vi "Run.vi"(8 "error in (no error)":errorcluster, 9 "Time Ratio used":dbl, 10 "Maze (0: Empty, -1: Enemy. >0: Teammate":i32[][](array[numeric]), 11 "Line Dancer in":refnum<class "Bricks.lvclass">) -> (0 "error out":errorcluster, 1 "Direction":T1, 2 "Action":T2, 3 "Line Dancer out":refnum<class "Bricks.lvclass">, 4 "Replicated":refnum<class "Square.lvclass">)   [LabVIEW 2015, in "Bricks.lvclass"]
uses:
  Bricks.lvclass
  Type Defs/Action Enum.ctl
  Type Defs/Direction Enum.ctl
  Square/Square.lvclass
  Common/Position.ctl
  Bricks.lvclass/Bricks.ctl
  Brick Wall Type.ctl
  SubVIs/Read-Only Globals.vi
  Common/Reverse Direction.vi
  Type Defs/SB Type Defs.lvlib
  Common/Common.lvlib
panel:
  # "NOTICE - YOU MUST NOT REMOVE THIS NOTICE. PER THE FOLLOWING LICENSE, YOU MAY REPRODUCE THIS SOFTWARE PROVIDED YOU FOLLOW THE TERMS\nOF THE LICENSE.\n\n---BEGIN BSD LICENSE (http://opensource.org/licenses/BSD-2-Clause)---\nCopyright (c) 2015, Endigit, Inc. <robert@endigit.com>\nAll rights reserved.\n\nRedistribution and use in source and binary forms, with or without modification, are permitted provided that the following conditions are met:\n\n1. Redistributions of source code must retain the above copyright notice, this list of conditions and the following disclaimer.\n\n2. Redistributions in binary form must reproduce the above copyright notice, this list of conditions and the following disclaimer in the documentation and/or other \nmaterials provided with the distribution.\n\nTHIS SOFTWARE IS PROVIDED BY THE COPYRIGHT HOLDERS AND CONTRIBUTORS \"AS IS\" AND ANY EXPRESS OR IMPLIED WARRANTIES, INCLUDING, BUT NOT \nLIMITED TO, THE IMPLIED WARRANTIES OF MERCHANTABILITY AND FITNESS FOR A PARTICULAR PURPOSE ARE DISCLAIMED. IN NO EVENT SHALL THE COPYRIGHT \nHOLDER OR CONTRIBUTORS BE LIABLE FOR ANY DIRECT, INDIRECT, INCIDENTAL, SPECIAL, EXEMPLARY, OR CONSEQUENTIAL DAMAGES (INCLUDING, BUT NOT \nLIMITED TO, PROCUREMENT OF SUBSTITUTE GOODS OR SERVICES; LOSS OF USE, DATA, OR PROFITS; OR BUSINESS INTERRUPTION) HOWEVER CAUSED AND ON \nANY THEORY OF LIABILITY, WHETHER IN CONTRACT, STRICT LIABILITY, OR TORT (INCLUDING NEGLIGENCE OR OTHERWISE) ARISING IN ANY WAY OUT OF THE USE \nOF THIS SOFTWARE, EVEN IF ADVISED OF THE POSSIBILITY OF SUCH DAMAGE.\n---END BSD LICENSE---"
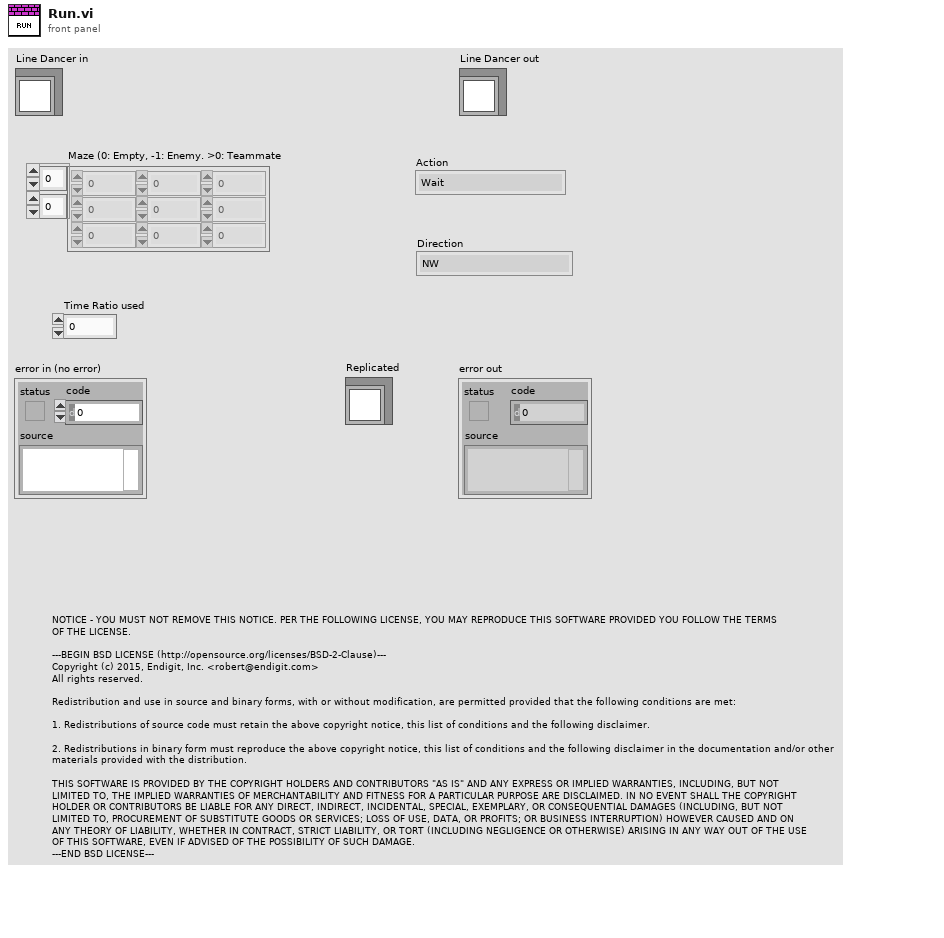
[diagram p1: front panel]
types:
  T1 = typedef "SB Type Defs.lvlib/Direction Enum.ctl" = enum16{"NW", "N", "NE", "E", "SE", "S", "SW", "W"}
  T2 = typedef "SB Type Defs.lvlib/Action Enum.ctl" = enum16{"Wait", "Move", "Attack", "Replicate"}
  T3 = typedef "Common.lvlib/Position.ctl" = cluster{"Column":i32, "Row":i32}
  T4 = typedef "Bricks.lvclass/Brick Wall Type.ctl" = enum16{"Starter", "Spawner", "Mason", "Wall", "Hottie"}
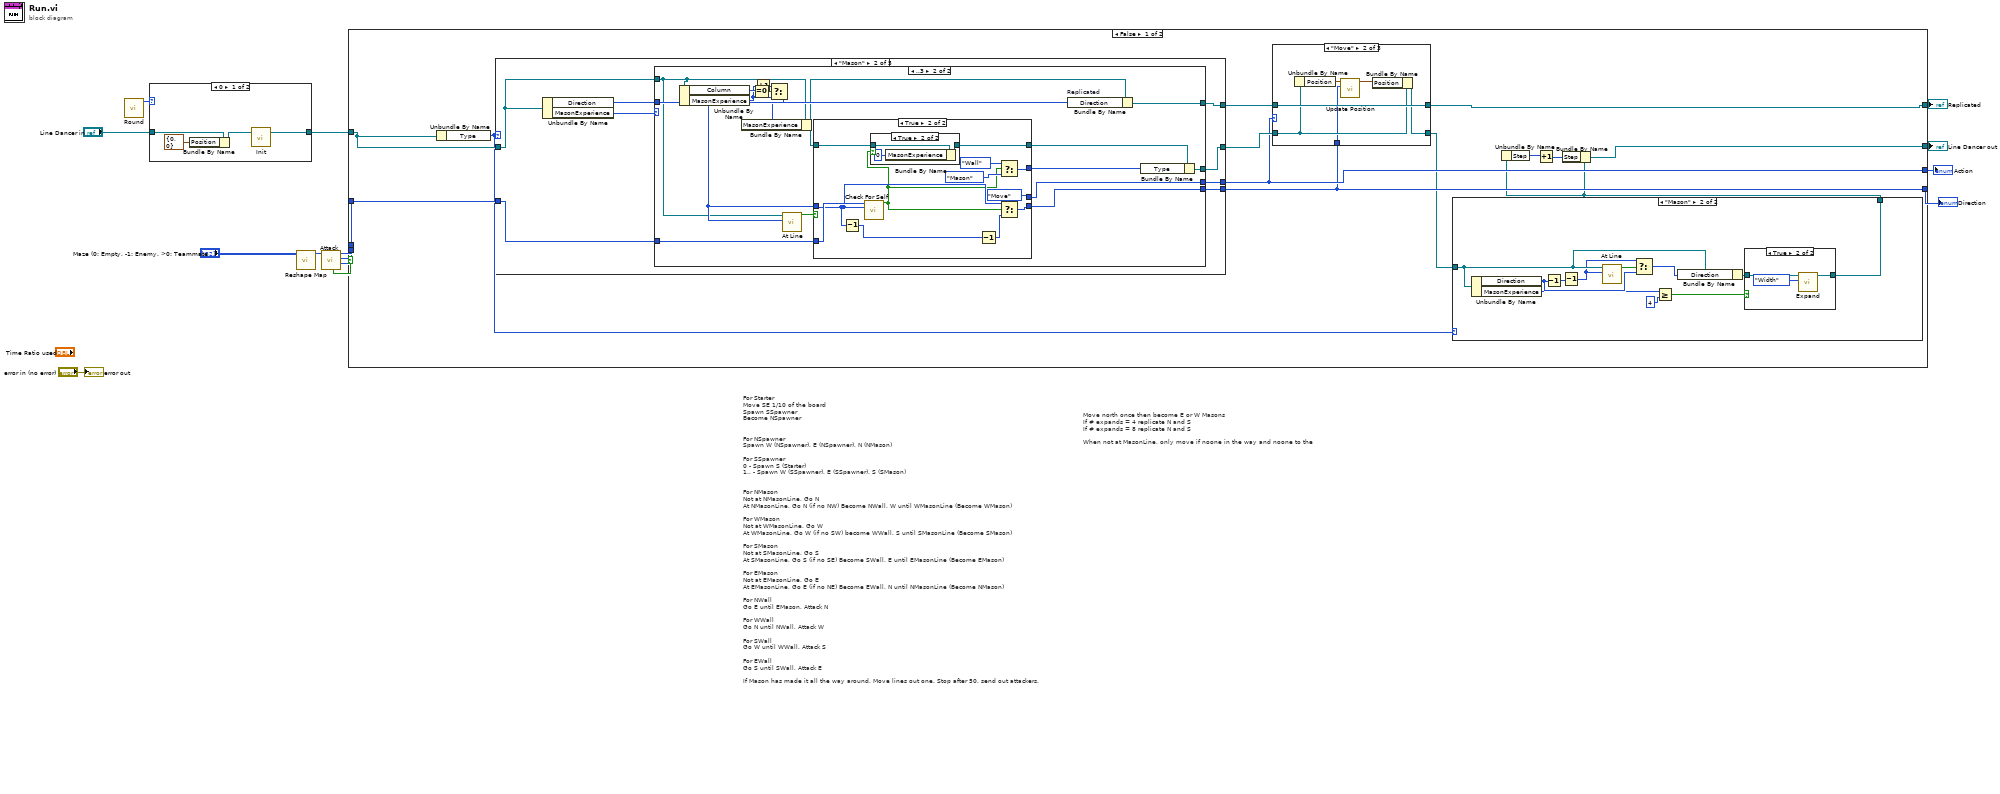
[diagram p0: block diagram]
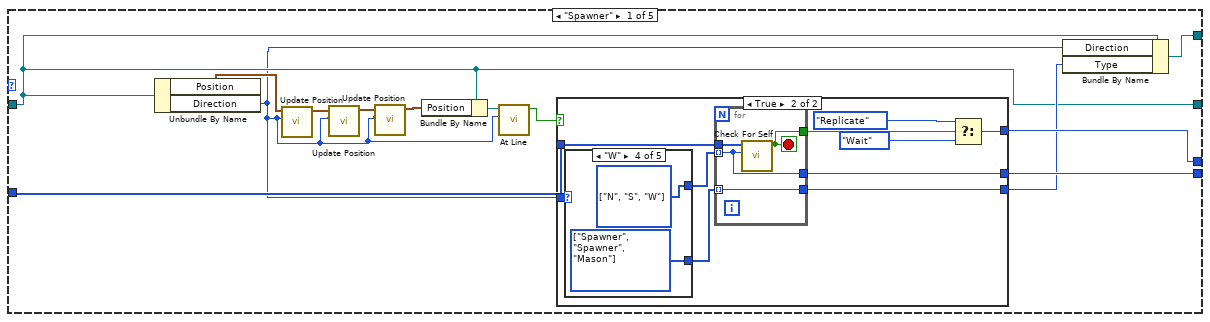
[diagram p5: hidden frame]
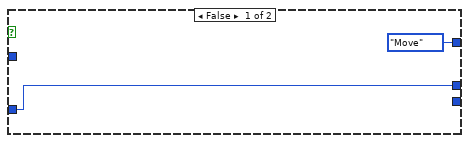
[diagram p6: hidden frame]
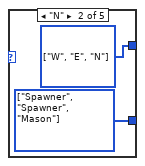
[diagram p8: hidden frame]
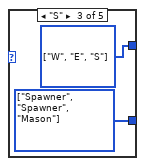
[diagram p9: hidden frame]
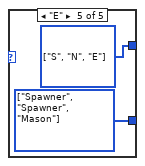
[diagram p10: hidden frame]
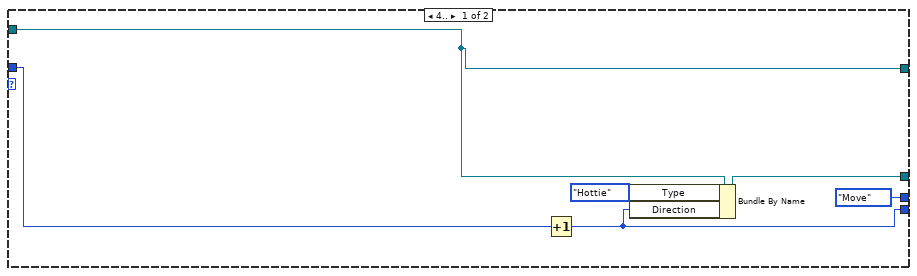
[diagram p11: hidden frame]
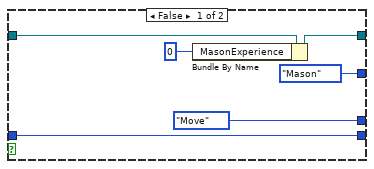
[diagram p12: hidden frame]
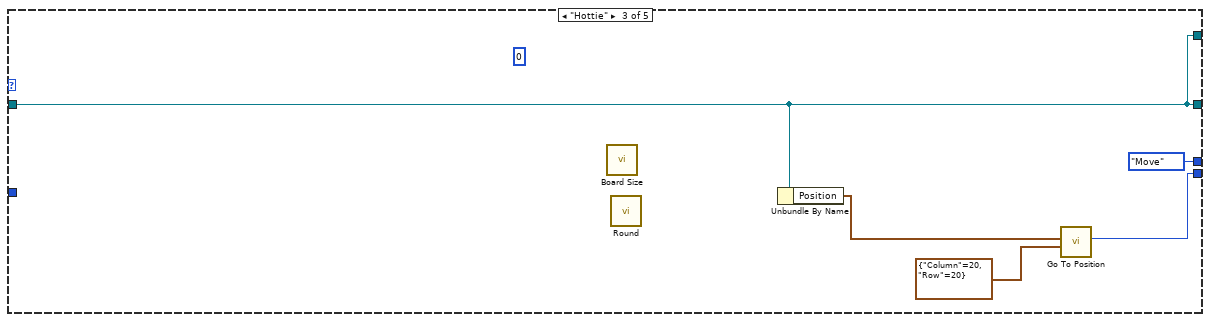
[diagram p14: hidden frame]
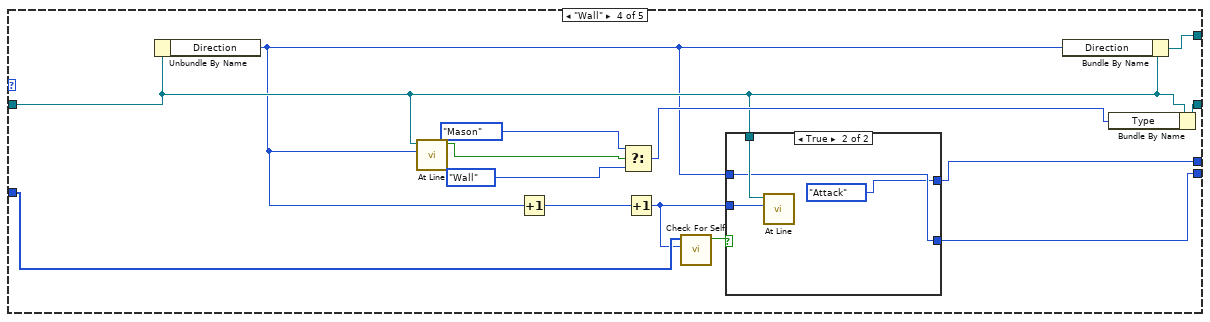
[diagram p15: hidden frame]
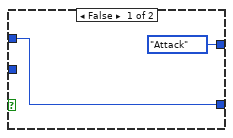
[diagram p16: hidden frame]
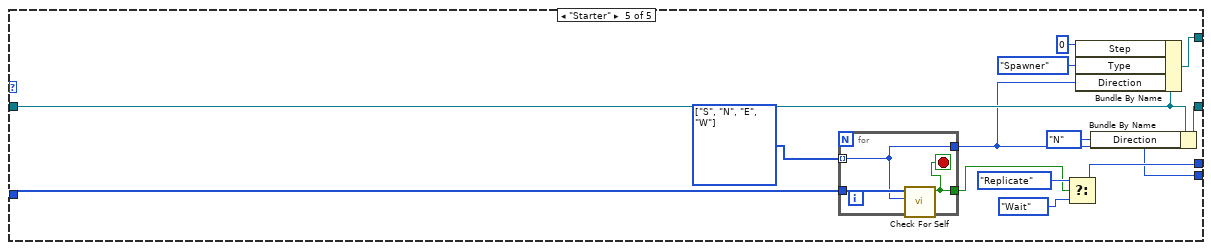
[diagram p17: hidden frame]
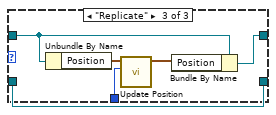
[diagram p19: hidden frame]
diagram:
  # "Move north once then become E or W Masons\nIf # expands = 4 replicate N and S\nIf # expands = 8 replicate N and S\n\nWhen not at MasonLine, only move if noone in the way and noone to the"
  # "For Starter \nMove SE 1/10 of the board\nSpawn SSpawner\nBecome NSpawner\n\n\nFor NSpawner\nSpawn W (NSpawner), E (NSpawner), N (NMason)\n\nFor SSpawner\n0 - Spawn S (Starter)\n1.. - Spawn W (SSpawner), E (SSpawner), S (SMason)\n\n\nFor NMason\nNot at NMasonLine, Go N\nAt NMasonLine, Go N (if no NW) Become NWall, W until WMasonLine (Become WMason)\n\nFor WMason\nNot at WMasonLine, Go W\nAt WMasonLine, Go W (if no SW) become WWall, S until SMasonLine (Become SMason)\n\nFor SMason\nNot at SMasonLine, Go S\nAt SMasonLine, Go S (if no SE) Become SWall, E until EMasonLine (Become EMason)\n\nFor EMason\nNot at EMasonLine, Go E\nAt EMasonLine, Go E (if no NE) Become EWall, N until NMasonLine (Become NMason)\n\nFor NWall\nGo E until EMason, Attack N\n\nFor WWall\nGo N until NWall, Attack W\n\nFor SWall\nGo W until WWall, Attack S\n\nFor EWall\nGo S until SWall, Attack E\n\nIf Mason has made it all the way around, Move lines out one. Stop after 50, send out attackers."
  n1 = call "Round.vi"() -> ("Round"=w1:i32)  [unwired: 11 in]
  n2 = case shown="0" w1 {
    tunnel: "Line Dancer in" -> [w18 w19]
    tunnel: [w17 w19] -> w2
    frame 0 {
      n3 = Bundle By Name(cluster=w18, "Position"=T3 {"Column"=0, "Row"=0}) -> (w16:refnum<class "Bricks.lvclass">)
      n4 = call "Init.vi"("Bricks in"=w16) -> ("Bricks out"=w17:refnum<class "Bricks.lvclass">)  [unwired: 10 in]
    }
    frame Default {
    }
  }
  n5 = call "Reshape Map.vi"("Maze (0: Empty, -1: Enemy. >0: Teammate"="Maze (0: Empty, -1: Enemy. >0: Teammate") -> ("Map"=w9:i32[])  [unwired: 9 in, 1 out]
  n6 = call "Attack.vi"("Maze (0: Empty, -1: Enemy. >0: Teammate"=w9) -> ("Direction"=w4:i32, "Action"=w5:T2, "Maze (0: Empty, -1: Enemy. >0: Teammate 2"=w7:i32[], "Enemy Found?"=w6:bool)  [unwired: 5 in, 2 out]
  n7 = case shown="False" w6 {
    tunnel: [w26 w194] -> w13
    tunnel: [w25 w193] -> w12
    tunnel: w2 -> [w32 w195]
    tunnel: [w29 w195] -> w11
    tunnel: [w20 w195] -> w10
    tunnel: w7 -> [w24 _]
    tunnel: w5 -> [_ w194]
    tunnel: w4 -> [_ w193]
    frame False {
      n8 = Unbundle By Name(w32) -> ("Type"=w23:T4)
      n9 = case shown="\"Mason\"" w23 {
        tunnel: [w59 w92 Action_Enum."Move" ("f") w148 w171] -> w26
        tunnel: [w60 w91 w138 w144 w167] -> w25
        tunnel: w24 -> [w61 w90 _ w147 w172]
        tunnel: [w58 w93 w141 w156 w174] -> w28
        tunnel: [w53 w89 w141 w154 w164] -> w27
        tunnel: w32 -> [w53 w87 w141 w150 w170]
        frame "Spawner" {
          n10 = Unbundle By Name(w53) -> ("Position"=w56:T3, "Direction"=w50:T1)
          n11 = call "Update Position.vi"("Direction"=w50, "Position in"=w56) -> ("Position out"=w55:T3)  [unwired: 9 in]
          n12 = call "Update Position.vi"("Direction"=w50, "Position in"=w55) -> ("Position out"=w54:T3)  [unwired: 9 in]
          n13 = call "Update Position.vi"("Direction"=w50, "Position in"=w54) -> ("Position out"=w51:T3)  [unwired: 9 in]
          n14 = Bundle By Name(cluster=w53, "Position"=w51) -> (w52:refnum<class "Bricks.lvclass">)
          n15 = call "At Line.vi"("Line"=w50, "Brick Wall in"=w52) -> ("At Line"=w49:bool)  [unwired: 9 in]
          n16 = case shown="True" w49 {
            tunnel: w61 -> [_ w73]
            tunnel: [w62 w72] -> w60
            tunnel: [Action_Enum."Move" ("f") w71] -> w59
            tunnel: [_ w70] -> w57
            tunnel: w50 -> [w62 w64]
            frame False {
            }
            frame True {
              n17 = case shown="\"W\"" w64 {
                tunnel: [_ w79 w81 w83 w85] -> w69
                tunnel: [_ w78 w80 w82 w84] -> w65
                frame Default {
                }
                frame "N" {
                  w78 = T4[] [enum."Spawner", enum."Spawner", enum."Mason"] items=["Starter", "Spawner", "Mason", "Wall", "Hottie"]
                  w79 = T1[] [enum."W", enum."E", enum."N"] items=["NW", "N", "NE", "E", "SE", "S", "SW", "W"]
                }
                frame "S" {
                  w80 = T4[] [enum."Spawner", enum."Spawner", enum."Mason"] items=["Starter", "Spawner", "Mason", "Wall", "Hottie"]
                  w81 = T1[] [enum."W", enum."E", enum."S"] items=["NW", "N", "NE", "E", "SE", "S", "SW", "W"]
                }
                frame "W" {
                  w82 = T4[] [enum."Spawner", enum."Spawner", enum."Mason"] items=["Starter", "Spawner", "Mason", "Wall", "Hottie"]
                  w83 = T1[] [enum."N", enum."S", enum."W"] items=["NW", "N", "NE", "E", "SE", "S", "SW", "W"]
                }
                frame "E" {
                  w84 = T4[] [enum."Spawner", enum."Spawner", enum."Mason"] items=["Starter", "Spawner", "Mason", "Wall", "Hottie"]
                  w85 = T1[] [enum."S", enum."N", enum."E"] items=["NW", "N", "NE", "E", "SE", "S", "SW", "W"]
                }
              }
              n18 = for {
                tunnel: w73 -> [w77]
                tunnel: w69 -> [w76] mode=indexing
                tunnel: [w76] -> w72
                tunnel: [w75] -> w68
                tunnel: w65 -> [w74] mode=indexing
                tunnel: [w74] -> w70
                stop <- w75 stop-if-true
                n19 = call "Check For Self.vi"("Direction"=w76, "Map"=w77) -> ("Clear?"=w75:bool)  [unwired: 9 in]
              }
              n20 = Select(t=Action_Enum."Replicate" ("f"), s=w68, f=Action_Enum."Wait") -> (s? t:f=w71:T2)
            }
          }
          n21 = Bundle By Name(cluster=w53, "Direction"=w50, "Type"=w57) -> (w58:refnum<class "Bricks.lvclass">)
        }
        frame "Mason" {
          n22 = Unbundle By Name(w87) -> ("Direction"=w88:T1, "MasonExperience"=w86:u8)
          n23 = case shown="..3" w86 {
            tunnel: [w97 w115] -> w93
            tunnel: [Action_Enum."Move" ("f") w113] -> w92
            tunnel: [w94 w112] -> w91
            tunnel: w90 -> [_ w111]
            tunnel: [w96 w110] -> w89
            tunnel: w88 -> [w98 w108]
            tunnel: w87 -> [w97 w106]
            frame 4.. {
              n24 = Increment(x=w98) -> (x+1=w94:T1)
              n25 = Bundle By Name(cluster=w97, "Type"=Brick_Wall_Type."Hottie" ("Player. Type"), "Direction"=w94) -> (w96:refnum<class "Bricks.lvclass">)
            }
            frame ..3 {
              n26 = Unbundle By Name(w106) -> ("Column"=w105:i32, "MasonExperience"=w103:u8)
              n27 = Equal To 0?(x=w105) -> (x = 0?=w104:bool)
              n28 = Increment(x=w103) -> (x+1=w102:u8)
              n29 = Select(t=w102, s=w104, f=w103) -> (s? t:f=w100:u8)
              n30 = Bundle By Name(cluster=w106, "MasonExperience"=w100) -> (w101:refnum<class "Bricks.lvclass">)
              n31 = call "At Line.vi"("Line"=w108, "Brick Wall in"=w106) -> ("At Line"=w114:bool)  [unwired: 9 in]
              n32 = case shown="True" w114 {
                tunnel: [Action_Enum."Move" ("f") Action_Enum."Move" ("f")] -> w113
                tunnel: [w120 w132] -> w112
                tunnel: w108 -> [w120 w131]
                tunnel: w111 -> [_ w133]
                tunnel: [Brick_Wall_Type."Mason" ("Player. Type") w126] -> w109
                tunnel: w101 -> [w118 w124]
                tunnel: [w117 w123] -> w107
                frame False {
                  n33 = Bundle By Name(cluster=w118, "MasonExperience"=u8 0) -> (w117:refnum<class "Bricks.lvclass">)
                }
                frame True {
                  n34 = Decrement(x=w131) -> (x-1=w130:T1)
                  n35 = call "Check For Self.vi"("Direction"=w131, "Map"=w133) -> ("Clear?"=w122:bool)  [unwired: 9 in]
                  n36 = case shown="True" w122 {
                    tunnel: w124 -> [w134 w137]
                    tunnel: [w134 w136] -> w123
                    frame False {
                    }
                    frame True {
                      n37 = Bundle By Name(cluster=w137, "MasonExperience"=u8 0) -> (w136:refnum<class "Bricks.lvclass">)
                    }
                  }
                  n38 = Decrement(x=w130) -> (x-1=w129:T1)
                  n39 = Select(t=Brick_Wall_Type."Wall", s=w122, f=Brick_Wall_Type."Mason" ("Player. Type")) -> (s? t:f=w126:T4)
                  n40 = Select(t=w131, s=w122, f=w129) -> (s? t:f=w132:T1)
                }
              }
              n41 = Bundle By Name "Replicated"(cluster=w101, "Direction"=w108) -> (w115:refnum<class "Bricks.lvclass">)
              n42 = Bundle By Name(cluster=w107, "Type"=w109) -> (w110:refnum<class "Bricks.lvclass">)
            }
          }
        }
        frame "Hottie" {
          (unwired) 0
          n43 = call "Board Size.vi"() -> ()  [unwired: 11 in, 1 out]
          n44 = call "Round.vi"() -> ()  [unwired: 11 in, 1 out]
          n45 = Unbundle By Name(w141) -> ("Position"=w140:T3)
          n46 = call "Go To Position.vi"("Target Position"=T3 {"Column"=20, "Row"=20}, "My Position"=w140) -> ("Direction"=w138:T1)  [unwired: 7 in, 2 out]
        }
        frame "Wall" {
          n47 = Unbundle By Name(w150) -> ("Direction"=w143:T1)
          n48 = call "At Line.vi"("Line"=w143, "Brick Wall in"=w150) -> ("At Line"=w155:bool)  [unwired: 9 in]
          n49 = Increment(x=w143) -> (x+1=w149:T1)
          n50 = Select(t=Brick_Wall_Type."Mason" ("Player. Type"), s=w155, f=Brick_Wall_Type."Wall" ("Player. Type")) -> (s? t:f=w151:T4)
          n51 = Increment(x=w149) -> (x+1=w146:T1)
          n52 = call "Check For Self.vi"("Direction"=w146, "Map"=w147) -> ("Clear?"=w145:bool)  [unwired: 9 in]
          n53 = case shown="True" w145 {
            tunnel: w150 -> [_ w162]
            tunnel: [Action_Enum."Attack" ("f") Action_Enum."Attack" ("f")] -> w148
            tunnel: w146 -> [_ w160]
            tunnel: [w157 w161] -> w144
            tunnel: w143 -> [w157 w161]
            frame False {
            }
            frame True {
              n54 = call "At Line.vi"("Line"=w160, "Brick Wall in"=w162) -> ()  [unwired: 9 in, 1 out]
            }
          }
          n55 = Bundle By Name(cluster=w150, "Direction"=w143) -> (w156:refnum<class "Bricks.lvclass">)
          n56 = Bundle By Name(cluster=w150, "Type"=w151) -> (w154:refnum<class "Bricks.lvclass">)
        }
        frame "Starter" {
          w168 = T1[] [enum."S", enum."N", enum."E", enum."W"] items=["NW", "N", "NE", "E", "SE", "S", "SW", "W"]
          n57 = for {
            tunnel: w172 -> [w178]
            tunnel: w168 -> [w176] mode=indexing
            tunnel: [w177] -> w165
            tunnel: [w176] -> w167
            stop <- w177 stop-if-true
            n58 = call "Check For Self.vi"("Direction"=w176, "Map"=w178) -> ("Clear?"=w177:bool)  [unwired: 9 in]
          }
          n59 = Select(t=Action_Enum."Replicate", s=w165, f=Action_Enum."Wait") -> (s? t:f=w171:T2)
          n60 = Bundle By Name(cluster=w170, "Step"=0, "Type"=Brick_Wall_Type."Spawner" ("Player Type"), "Direction"=w167) -> (w174:refnum<class "Bricks.lvclass">)
          n61 = Bundle By Name(cluster=w170, "Direction"=Direction_Enum."N" ("Player.Direction")) -> (w164:refnum<class "Bricks.lvclass">)
        }
      }
      n62 = case shown="\"Move\"" w26 {
        tunnel: w28 -> [w180 w186 w189]
        tunnel: [w180 w186 w188] -> w20
        tunnel: w27 -> [w179 w185 w187]
        tunnel: [w179 w183 w187] -> w22
        tunnel: w25 -> [_ w181 w190]
        frame Default {
        }
        frame "Move" {
          n63 = Unbundle By Name(w185) -> ("Position"=w184:T3)
          n64 = call "Update Position.vi"("Direction"=w181, "Position in"=w184) -> ("Position out"=w182:T3)  [unwired: 9 in]
          n65 = Bundle By Name(cluster=w185, "Position"=w182) -> (w183:refnum<class "Bricks.lvclass">)
        }
        frame "Replicate" {
          n66 = Unbundle By Name(w189) -> ("Position"=w192:T3)
          n67 = call "Update Position.vi"("Direction"=w190, "Position in"=w192) -> ("Position out"=w191:T3)  [unwired: 9 in]
          n68 = Bundle By Name(cluster=w189, "Position"=w191) -> (w188:refnum<class "Bricks.lvclass">)
        }
      }
      n69 = case shown="\"Mason\"" w23 {
        tunnel: w22 -> [w33 w43]
        tunnel: [w33 w35] -> w21
        frame Default {
        }
        frame "Mason" {
          n70 = Unbundle By Name(w43) -> ("Direction"=w41:T1, "MasonExperience"=w37:u8)
          n71 = Decrement(x=w41) -> (x-1=w44:T1)
          n72 = Decrement(x=w44) -> (x-1=w40:T1)
          n73 = call "At Line.vi"("Line"=w40, "Brick Wall in"=w43) -> ("At Line"=w38:bool)  [unwired: 9 in]
          n74 = Select(t=w40, s=w38, f=w41) -> (s? t:f=w42:T1)
          n75 = Greater Or Equal?(x=w37, y=u8 4) -> (x >= y?=w34:bool)
          n76 = Bundle By Name(cluster=w43, "Direction"=w42) -> (w39:refnum<class "Bricks.lvclass">)
          n77 = case shown="True" w34 {
            tunnel: w39 -> [w45 w48]
            tunnel: [w45 w47] -> w35
            frame False {
            }
            frame True {
              n78 = call-dynamic "Expand.vi"("Expand Direction"=enum16{"Height", "Width", "Both"}."Width", "Brick Wall in"=w48) -> ("Brick Wall out"=w47:refnum<class "Bricks.lvclass">)  [unwired: 8 in, 1 out]
            }
          }
        }
      }
      n79 = Unbundle By Name(w21) -> ("Step"=w31:i32)
      n80 = Increment(x=w31) -> (x+1=w30:i32)
      n81 = Bundle By Name(cluster=w21, "Step"=w30) -> (w29:refnum<class "Bricks.lvclass">)
    }
    frame True {
    }
  }
  "Line Dancer out" <- w11
  "Action" <- w13
  "Direction" <- w12
  "Replicated" <- w10
  "error out" <- "error in (no error)"
